vi "Analysis Vol. 3 CSV Read.vi"() -> ()   [LabVIEW 2014] (continued)
2399.01, 2394.29, 2389.45, 2384.42, 2379.46, 2374.5, 2369.85, 2365.32, 2360.97, 2356.55, 2352.38, 2348.17, 2343.81, 2339.36, 2334.89, 2330.02, 2324.83, 2319.71, 2314.4, 2308.87, 2303.33, 2297.78, 2291.87, 2285.95, 2280.16, 2274.42, 2268.74, 2263.33, 2257.96, 2252.44, 2246.89, 2241.34, 2235.57, 2229.67, 2223.7, 2217.56, 2211.19, 2204.8, 2198.33, 2191.78, 2185.2, 2178.68, 2172.08, 2165.53, 2159.12, 2152.93, 2146.84, 2140.86, 2134.88, 2128.82, 2122.54, 2116.07, 2109.39, 2102.62, 2095.88, 2089.08, 2082.34, 2075.72, 2068.95, 2061.64, 2053.63, 2044.73, 2034.67, 2023.62, 2011.78, 1999.41, 1987.03, 1974.65, 1962.27, 1949.9, 1937.52]}, {"Y"=[4.0, 5.0, 6.0, 7.0, 8.0, 9.0, 10.0, 11.0, 12.0, 13.0, 14.0, 15.0, 16.0, 17.0, 18.0, 19.0, 20.0, 21.0, 22.0, 23.0, 24.0, 25.0, 26.0, 27.0, 28.0, 29.0, 30.0, 31.0, 32.0, 33.0, 34.0, 35.0, 36.0, 37.0, 38.0, 39.0, 40.0, 41.0, 42.0, 43.0, 44.0, 45.0, 46.0, 47.0, 48.0, 49.0, 50.0, 51.0, 52.0, 53.0, 54.0, 55.0, 56.0, 57.0, 58.0, 59.0, 60.0, 61.0, 62.0, 63.0, 64.0, 65.0, 66.0, 67.0, 68.0, 69.0, 70.0, 71.0, 72.0, 73.0, 74.0, 75.0, 76.0, 77.0, 78.0, 79.0, 80.0, 81.0, 82.0, 83.0, 84.0, 85.0, 86.0, 87.0, 88.0, 89.0, 90.0, 91.0, 92.0, 93.0, 94.0, 95.0], "Y"=[2494.33, 2488.95, 2483.63, 2478.55, 2473.6, 2468.64, 2463.81, 2458.93, 2454.17, 2449.41, 2444.68, 2439.89, 2435.11, 2430.15, 2425.39, 2420.72, 2416.24, 2411.89, 2407.71, 2403.39, 2399.01, 2394.29, 2389.45, 2384.42, 2379.46, 2374.5, 2369.85, 2365.32, 2360.97, 2356.55, 2352.38, 2348.17, 2343.81, 2339.36, 2334.89, 2330.02, 2324.83, 2319.71, 2314.4, 2308.87, 2303.33, 2297.78, 2291.87, 2285.95, 2280.16, 2274.42, 2268.74, 2263.33, 2257.96, 2252.44, 2246.89, 2241.34, 2235.57, 2229.67, 2223.7, 2217.56, 2211.19, 2204.8, 2198.33, 2191.78, 2185.2, 2178.68, 2172.08, 2165.53, 2159.12, 2152.93, 2146.84, 2140.86, 2134.88, 2128.82, 2122.54, 2116.07, 2109.39, 2102.62, 2095.88, 2089.08, 2082.34, 2075.72, 2068.95, 2061.64, 2053.63, 2044.73, 2034.67, 2023.62, 2011.78, 1999.41, 1987.03, 1974.65, 1962.27, 1949.9, 1937.52]}, {"Y"=[4.0, 5.0, 6.0, 7.0, 8.0, 9.0, 10.0, 11.0, 12.0, 13.0, 14.0, 15.0, 16.0, 17.0, 18.0, 19.0, 20.0, 21.0, 22.0, 23.0, 24.0, 25.0, 26.0, 27.0, 28.0, 29.0, 30.0, 31.0, 32.0, 33.0, 34.0, 35.0, 36.0, 37.0, 38.0, 39.0, 40.0, 41.0, 42.0, 43.0, 44.0, 45.0, 46.0, 47.0, 48.0, 49.0, 50.0, 51.0, 52.0, 53.0, 54.0, 55.0, 56.0, 57.0, 58.0, 59.0, 60.0, 61.0, 62.0, 63.0, 64.0, 65.0, 66.0, 67.0, 68.0, 69.0, 70.0, 71.0, 72.0, 73.0, 74.0, 75.0, 76.0, 77.0, 78.0, 79.0, 80.0, 81.0, 82.0, 83.0, 84.0, 85.0, 86.0, 87.0, 88.0, 89.0, 90.0, 91.0, 92.0, 93.0, 94.0, 95.0], "Y"=[2494.33, 2488.95, 2483.63, 2478.55, 2473.6, 2468.64, 2463.81, 2458.93, 2454.17, 2449.41, 2444.68, 2439.89, 2435.11, 2430.15, 2425.39, 2420.72, 2416.24, 2411.89, 2407.71, 2403.39, 2399.01, 2394.29, 2389.45, 2384.42, 2379.46, 2374.5, 2369.85, 2365.32, 2360.97, 2356.55, 2352.38, 2348.17, 2343.81, 2339.36, 2334.89, 2330.02, 2324.83, 2319.71, 2314.4, 2308.87, 2303.33, 2297.78, 2291.87, 2285.95, 2280.16, 2274.42, 2268.74, 2263.33, 2257.96, 2252.44, 2246.89, 2241.34, 2235.57, 2229.67, 2223.7, 2217.56, 2211.19, 2204.8, 2198.33, 2191.78, 2185.2, 2178.68, 2172.08, 2165.53, 2159.12, 2152.93, 2146.84, 2140.86, 2134.88, 2128.82, 2122.54, 2116.07, 2109.39, 2102.62, 2095.88, 2089.08, 2082.34, 2075.72, 2068.95, 2061.64, 2053.63, 2044.73, 2034.67, 2023.62, 2011.78, 1999.41, 1987.03, 1974.65, 1962.27, 1949.9, 1937.52]}, {"Y"=[4.0, 5.0, 6.0, 7.0, 8.0, 9.0, 10.0, 11.0, 12.0, 13.0, 14.0, 15.0, 16.0, 17.0, 18.0, 19.0, 20.0, 21.0, 22.0, 23.0, 24.0, 25.0, 26.0, 27.0, 28.0, 29.0, 30.0, 31.0, 32.0, 33.0, 34.0, 35.0, 36.0, 37.0, 38.0, 39.0, 40.0, 41.0, 42.0, 43.0, 44.0, 45.0, 46.0, 47.0, 48.0, 49.0, 50.0, 51.0, 52.0, 53.0, 54.0, 55.0, 56.0, 57.0, 58.0, 59.0, 60.0, 61.0, 62.0, 63.0, 64.0, 65.0, 66.0, 67.0, 68.0, 69.0, 70.0, 71.0, 72.0, 73.0, 74.0, 75.0, 76.0, 77.0, 78.0, 79.0, 80.0, 81.0, 82.0, 83.0, 84.0, 85.0, 86.0, 87.0, 88.0, 89.0, 90.0, 91.0, 92.0, 93.0, 94.0, 95.0], "Y"=[2494.33, 2488.95, 2483.63, 2478.55, 2473.6, 2468.64, 2463.81, 2458.93, 2454.17, 2449.41, 2444.68, 2439.89, 2435.11, 2430.15, 2425.39, 2420.72, 2416.24, 2411.89, 2407.71, 2403.39, 2399.01, 2394.29, 2389.45, 2384.42, 2379.46, 2374.5, 2369.85, 2365.32, 2360.97, 2356.55, 2352.38, 2348.17, 2343.81, 2339.36, 2334.89, 2330.02, 2324.83, 2319.71, 2314.4, 2308.87, 2303.33, 2297.78, 2291.87, 2285.95, 2280.16, 2274.42, 2268.74, 2263.33, 2257.96, 2252.44, 2246.89, 2241.34, 2235.57, 2229.67, 2223.7, 2217.56, 2211.19, 2204.8, 2198.33, 2191.78, 2185.2, 2178.68, 2172.08, 2165.53, 2159.12, 2152.93, 2146.84, 2140.86, 2134.88, 2128.82, 2122.54, 2116.07, 2109.39, 2102.62, 2095.88, 2089.08, 2082.34, 2075.72, 2068.95, 2061.64, 2053.63, 2044.73, 2034.67, 2023.62, 2011.78, 1999.41, 1987.03, 1974.65, 1962.27, 1949.9, 1937.52]}, {"Y"=[4.0, 5.0, 6.0, 7.0, 8.0, 9.0, 10.0, 11.0, 12.0, 13.0, 14.0, 15.0, 16.0, 17.0, 18.0, 19.0, 20.0, 21.0, 22.0, 23.0, 24.0, 25.0, 26.0, 27.0, 28.0, 29.0, 30.0, 31.0, 32.0, 33.0, 34.0, 35.0, 36.0, 37.0, 38.0, 39.0, 40.0, 41.0, 42.0, 43.0, 44.0, 45.0, 46.0, 47.0, 48.0, 49.0, 50.0, 51.0, 52.0, 53.0, 54.0, 55.0, 56.0, 57.0, 58.0, 59.0, 60.0, 61.0, 62.0, 63.0, 64.0, 65.0, 66.0, 67.0, 68.0, 69.0, 70.0, 71.0, 72.0, 73.0, 74.0, 75.0, 76.0, 77.0, 78.0, 79.0, 80.0, 81.0, 82.0, 83.0, 84.0, 85.0, 86.0, 87.0, 88.0, 89.0, 90.0, 91.0, 92.0, 93.0, 94.0, 95.0], "Y"=[2494.33, 2488.95, 2483.63, 2478.55, 2473.6, 2468.64, 2463.81, 2458.93, 2454.17, 2449.41, 2444.68, 2439.89, 2435.11, 2430.15, 2425.39, 2420.72, 2416.24, 2411.89, 2407.71, 2403.39, 2399.01, 2394.29, 2389.45, 2384.42, 2379.46, 2374.5, 2369.85, 2365.32, 2360.97, 2356.55, 2352.38, 2348.17, 2343.81, 2339.36, 2334.89, 2330.02, 2324.83, 2319.71, 2314.4, 2308.87, 2303.33, 2297.78, 2291.87, 2285.95, 2280.16, 2274.42, 2268.74, 2263.33, 2257.96, 2252.44, 2246.89, 2241.34, 2235.57, 2229.67, 2223.7, 2217.56, 2211.19, 2204.8, 2198.33, 2191.78, 2185.2, 2178.68, 2172.08, 2165.53, 2159.12, 2152.93, 2146.84, 2140.86, 2134.88, 2128.82, 2122.54, 2116.07, 2109.39, 2102.62, 2095.88, 2089.08, 2082.34, 2075.72, 2068.95, 2061.64, 2053.63, 2044.73, 2034.67, 2023.62, 2011.78, 1999.41, 1987.03, 1974.65, 1962.27, 1949.9, 1937.52]}, {"Y"=[4.0, 5.0, 6.0, 7.0, 8.0, 9.0, 10.0, 11.0, 12.0, 13.0, 14.0, 15.0, 16.0, 17.0, 18.0, 19.0, 20.0, 21.0, 22.0, 23.0, 24.0, 25.0, 26.0, 27.0, 28.0, 29.0, 30.0, 31.0, 32.0, 33.0, 34.0, 35.0, 36.0, 37.0, 38.0, 39.0, 40.0, 41.0, 42.0, 43.0, 44.0, 45.0, 46.0, 47.0, 48.0, 49.0, 50.0, 51.0, 52.0, 53.0, 54.0, 55.0, 56.0, 57.0, 58.0, 59.0, 60.0, 61.0, 62.0, 63.0, 64.0, 65.0, 66.0, 67.0, 68.0, 69.0, 70.0, 71.0, 72.0, 73.0, 74.0, 75.0, 76.0, 77.0, 78.0, 79.0, 80.0, 81.0, 82.0, 83.0, 84.0, 85.0, 86.0, 87.0, 88.0, 89.0, 90.0, 91.0, 92.0, 93.0, 94.0, 95.0], "Y"=[2494.33, 2488.95, 2483.63, 2478.55, 2473.6, 2468.64, 2463.81, 2458.93, 2454.17, 2449.41, 2444.68, 2439.89, 2435.11, 2430.15, 2425.39, 2420.72, 2416.24, 2411.89, 2407.71, 2403.39, 2399.01, 2394.29, 2389.45, 2384.42, 2379.46, 2374.5, 2369.85, 2365.32, 2360.97, 2356.55, 2352.38, 2348.17, 2343.81, 2339.36, 2334.89, 2330.02, 2324.83, 2319.71, 2314.4, 2308.87, 2303.33, 2297.78, 2291.87, 2285.95, 2280.16, 2274.42, 2268.74, 2263.33, 2257.96, 2252.44, 2246.89, 2241.34, 2235.57, 2229.67, 2223.7, 2217.56, 2211.19, 2204.8, 2198.33, 2191.78, 2185.2, 2178.68, 2172.08, 2165.53, 2159.12, 2152.93, 2146.84, 2140.86, 2134.88, 2128.82, 2122.54, 2116.07, 2109.39, 2102.62, 2095.88, 2089.08, 2082.34, 2075.72, 2068.95, 2061.64, 2053.63, 2044.73, 2034.67, 2023.62, 2011.78, 1999.41, 1987.03, 1974.65, 1962.27, 1949.9, 1937.52]}, {"Y"=[4.0, 5.0, 6.0, 7.0, 8.0, 9.0, 10.0, 11.0, 12.0, 13.0, 14.0, 15.0, 16.0, 17.0, 18.0, 19.0, 20.0, 21.0, 22.0, 23.0, 24.0, 25.0, 26.0, 27.0, 28.0, 29.0, 30.0, 31.0, 32.0, 33.0, 34.0, 35.0, 36.0, 37.0, 38.0, 39.0, 40.0, 41.0, 42.0, 43.0, 44.0, 45.0, 46.0, 47.0, 48.0, 49.0, 50.0, 51.0, 52.0, 53.0, 54.0, 55.0, 56.0, 57.0, 58.0, 59.0, 60.0, 61.0, 62.0, 63.0, 64.0, 65.0, 66.0, 67.0, 68.0, 69.0, 70.0, 71.0, 72.0, 73.0, 74.0, 75.0, 76.0, 77.0, 78.0, 79.0, 80.0, 81.0, 82.0, 83.0, 84.0, 85.0, 86.0, 87.0, 88.0, 89.0, 90.0, 91.0, 92.0, 93.0, 94.0, 95.0], "Y"=[2494.33, 2488.95, 2483.63, 2478.55, 2473.6, 2468.64, 2463.81, 2458.93, 2454.17, 2449.41, 2444.68, 2439.89, 2435.11, 2430.15, 2425.39, 2420.72, 2416.24, 2411.89, 2407.71, 2403.39, 2399.01, 2394.29, 2389.45, 2384.42, 2379.46, 2374.5, 2369.85, 2365.32, 2360.97, 2356.55, 2352.38, 2348.17, 2343.81, 2339.36, 2334.89, 2330.02, 2324.83, 2319.71, 2314.4, 2308.87, 2303.33, 2297.78, 2291.87, 2285.95, 2280.16, 2274.42, 2268.74, 2263.33, 2257.96, 2252.44, 2246.89, 2241.34, 2235.57, 2229.67, 2223.7, 2217.56, 2211.19, 2204.8, 2198.33, 2191.78, 2185.2, 2178.68, 2172.08, 2165.53, 2159.12, 2152.93, 2146.84, 2140.86, 2134.88, 2128.82, 2122.54, 2116.07, 2109.39, 2102.62, 2095.88, 2089.08, 2082.34, 2075.72, 2068.95, 2061.64, 2053.63, 2044.73, 2034.67, 2023.62, 2011.78, 1999.41, 1987.03, 1974.65, 1962.27, 1949.9, 1937.52]}, {"Y"=[4.0, 5.0, 6.0, 7.0, 8.0, 9.0, 10.0, 11.0, 12.0, 13.0, 14.0, 15.0, 16.0, 17.0, 18.0, 19.0, 20.0, 21.0, 22.0, 23.0, 24.0, 25.0, 26.0, 27.0, 28.0, 29.0, 30.0, 31.0, 32.0, 33.0, 34.0, 35.0, 36.0, 37.0, 38.0, 39.0, 40.0, 41.0, 42.0, 43.0, 44.0, 45.0, 46.0, 47.0, 48.0, 49.0, 50.0, 51.0, 52.0, 53.0, 54.0, 55.0, 56.0, 57.0, 58.0, 59.0, 60.0, 61.0, 62.0, 63.0, 64.0, 65.0, 66.0, 67.0, 68.0, 69.0, 70.0, 71.0, 72.0, 73.0, 74.0, 75.0, 76.0, 77.0, 78.0, 79.0, 80.0, 81.0, 82.0, 83.0, 84.0, 85.0, 86.0, 87.0, 88.0, 89.0, 90.0, 91.0, 92.0, 93.0, 94.0, 95.0], "Y"=[2494.33, 2488.95, 2483.63, 2478.55, 2473.6, 2468.64, 2463.81, 2458.93, 2454.17, 2449.41, 2444.68, 2439.89, 2435.11, 2430.15, 2425.39, 2420.72, 2416.24, 2411.89, 2407.71, 2403.39, 2399.01, 2394.29, 2389.45, 2384.42, 2379.46, 2374.5, 2369.85, 2365.32, 2360.97, 2356.55, 2352.38, 2348.17, 2343.81, 2339.36, 2334.89, 2330.02, 2324.83, 2319.71, 2314.4, 2308.87, 2303.33, 2297.78, 2291.87, 2285.95, 2280.16, 2274.42, 2268.74, 2263.33, 2257.96, 2252.44, 2246.89, 2241.34, 2235.57, 2229.67, 2223.7, 2217.56, 2211.19, 2204.8, 2198.33, 2191.78, 2185.2, 2178.68, 2172.08, 2165.53, 2159.12, 2152.93, 2146.84, 2140.86, 2134.88, 2128.82, 2122.54, 2116.07, 2109.39, 2102.62, 2095.88, 2089.08, 2082.34, 2075.72, 2068.95, 2061.64, 2053.63, 2044.73, 2034.67, 2023.62, 2011.78, 1999.41, 1987.03, 1974.65, 1962.27, 1949.9, 1937.52]}] caption="Reference plot:"
  in  "Load Dye 2":path=path "C:/Users/labuser/Desktop/Arbeit/Experimental Data/Selection via Gelation Project/2021-05-10 Dorothea meltingcurves/melting curves dna/step 1/melting curves 2021-05-12 -  Melt Curve RFU Results_FAM.csv"
  in  "Reference \non/off":bool=TRUE
  in  "STOP":bool
  out "Dye2withBaselineCorrectio":dbl[][](array[numeric])=[[0.0, 4721.59401069584, 4726.64557983141, 4731.69720585736, 4736.72035903032, 4741.6216490146, 4746.19464965707, 4750.77546264608, 4755.13221756768, 4759.44159755608, 4763.89791396376, 4768.45333576223, 4773.03439707822, 4777.77977396049, 4782.53780205103, 4787.25892226452, 4791.97529358062, 4796.91300937426, 4801.61522170524, 4806.32202250741, 4810.93165344366, 4815.32270660079, 4819.15747599548, 4823.15365637635, 4827.05620435302, 4831.11932397294, 4835.44455829981, 4840.13821284811, 4844.89868237613, 4849.72347270819, 4854.55598974164, 4859.30049974853, 4863.79330506012, 4868.06003683746, 4872.40360247469, 4876.48257410991, 4880.49222398608, 4884.66860430045, 4889.23532566947, 4893.60767815332, 4898.14721099649, 4902.8335972453, 4907.55580598647, 4911.69484044918, 4915.77151333199, 4919.86201149958, 4923.86627488786, 4927.85737755496, 4932.2086278581, 4936.7058924887, 4941.19259968617, 4945.45646686776, 4949.70852542204, 4954.02738779181, 4958.70620656545, 4963.3373268874, 4968.1270371998, 4972.78255793418, 4977.19752478803, 4980.86104806113, 4984.48505580278, 4988.14503964276, 4991.90606946941, 4995.71108454377, 4999.84169025866, 5003.79220065297, 5007.79451836246, 5011.69904254421, 5015.55248715627, 5019.4211520663, 5023.46854922211, 5027.31444684709, 5031.28390945256, 5035.21630010117, 5039.18771534215, 5043.297928556, 5047.28534502707, 5050.97484453209, 5054.58029400532, 5057.9925558248, 5061.03113489723, 5064.19189460972, 5067.37675898951, 5070.55704176141, 5073.65523291141, 5076.76172826201, 5079.69065606831, 5082.68394797735, 5085.57389782356, 5088.5962155605, 5091.68654322026, 5094.89447116713, 5098.12219561475, 5101.43434995644, 5104.58157320642, 5107.8598516264, 5111.36204846851, 5114.81342414506, 5118.78218391394, 5123.03726144675, 5127.41177098768, 5131.74312272957, 5136.39151578824, 5140.39791781123, 5144.63135682615, 5148.75170796368, 5152.93125959229, 5157.09173855716, 5161.70979771955, 5166.02742357914, 5170.41958302151, 5174.69823644507, 5178.76165176852, 5182.86433598839, 5187.08415587395, 5191.40660982161, 5195.97381163606, 5200.69896363319, 5205.2834506216, 5209.82139171157, 5214.016470183, 5217.77454547304, 5221.28564607111, 5224.59798553874, 5227.60049882735, 5230.48504907438, 5233.03480180081, 5235.09586969891]]
  # "Load data in a defined format:"
  # "Data Format:\n* 1st column contain Temperature/Time\n* all the rest columns contain signal of samples"
  # "Select wells, give names, and define concentrations:"
  # "Minutes"
  # "Temperature"
  # "divide all channels by reference channel"
  # "dbr=divided by reference"
  # "nr=no reference"
  # "Graph3 - Michaelis-Menten\n(Needs a fit from Graph2)"
  # "Graph1: Data (+/- ref correction)"
  # "Graph2: Corrections & fits"
  # "(Needs Baseline)"
  # "(Needs Concentrations)"
  # "Vmax"
  # "Km"
  # "Graph4: Turnover Analysis\n(Needs line fit in plateau in Graph2 to adjust concentration)"
  # "Graph3 - Michaelis-Menten\n(Needs a fit from Graph2)"
  # "Graph1: Data (+/- ref correction)"
  # "Graph2: Corrections & fits"
  # "(Needs Baseline)"
  # "(Needs Concentrations)"
  # "Vmax"
  # "Km"
  # "Intercalator"
  # "Quenching"
  # "R=0.0019872041 kcal/(mole*K)"
  # "Constant Concentration"
  # "Dilution"
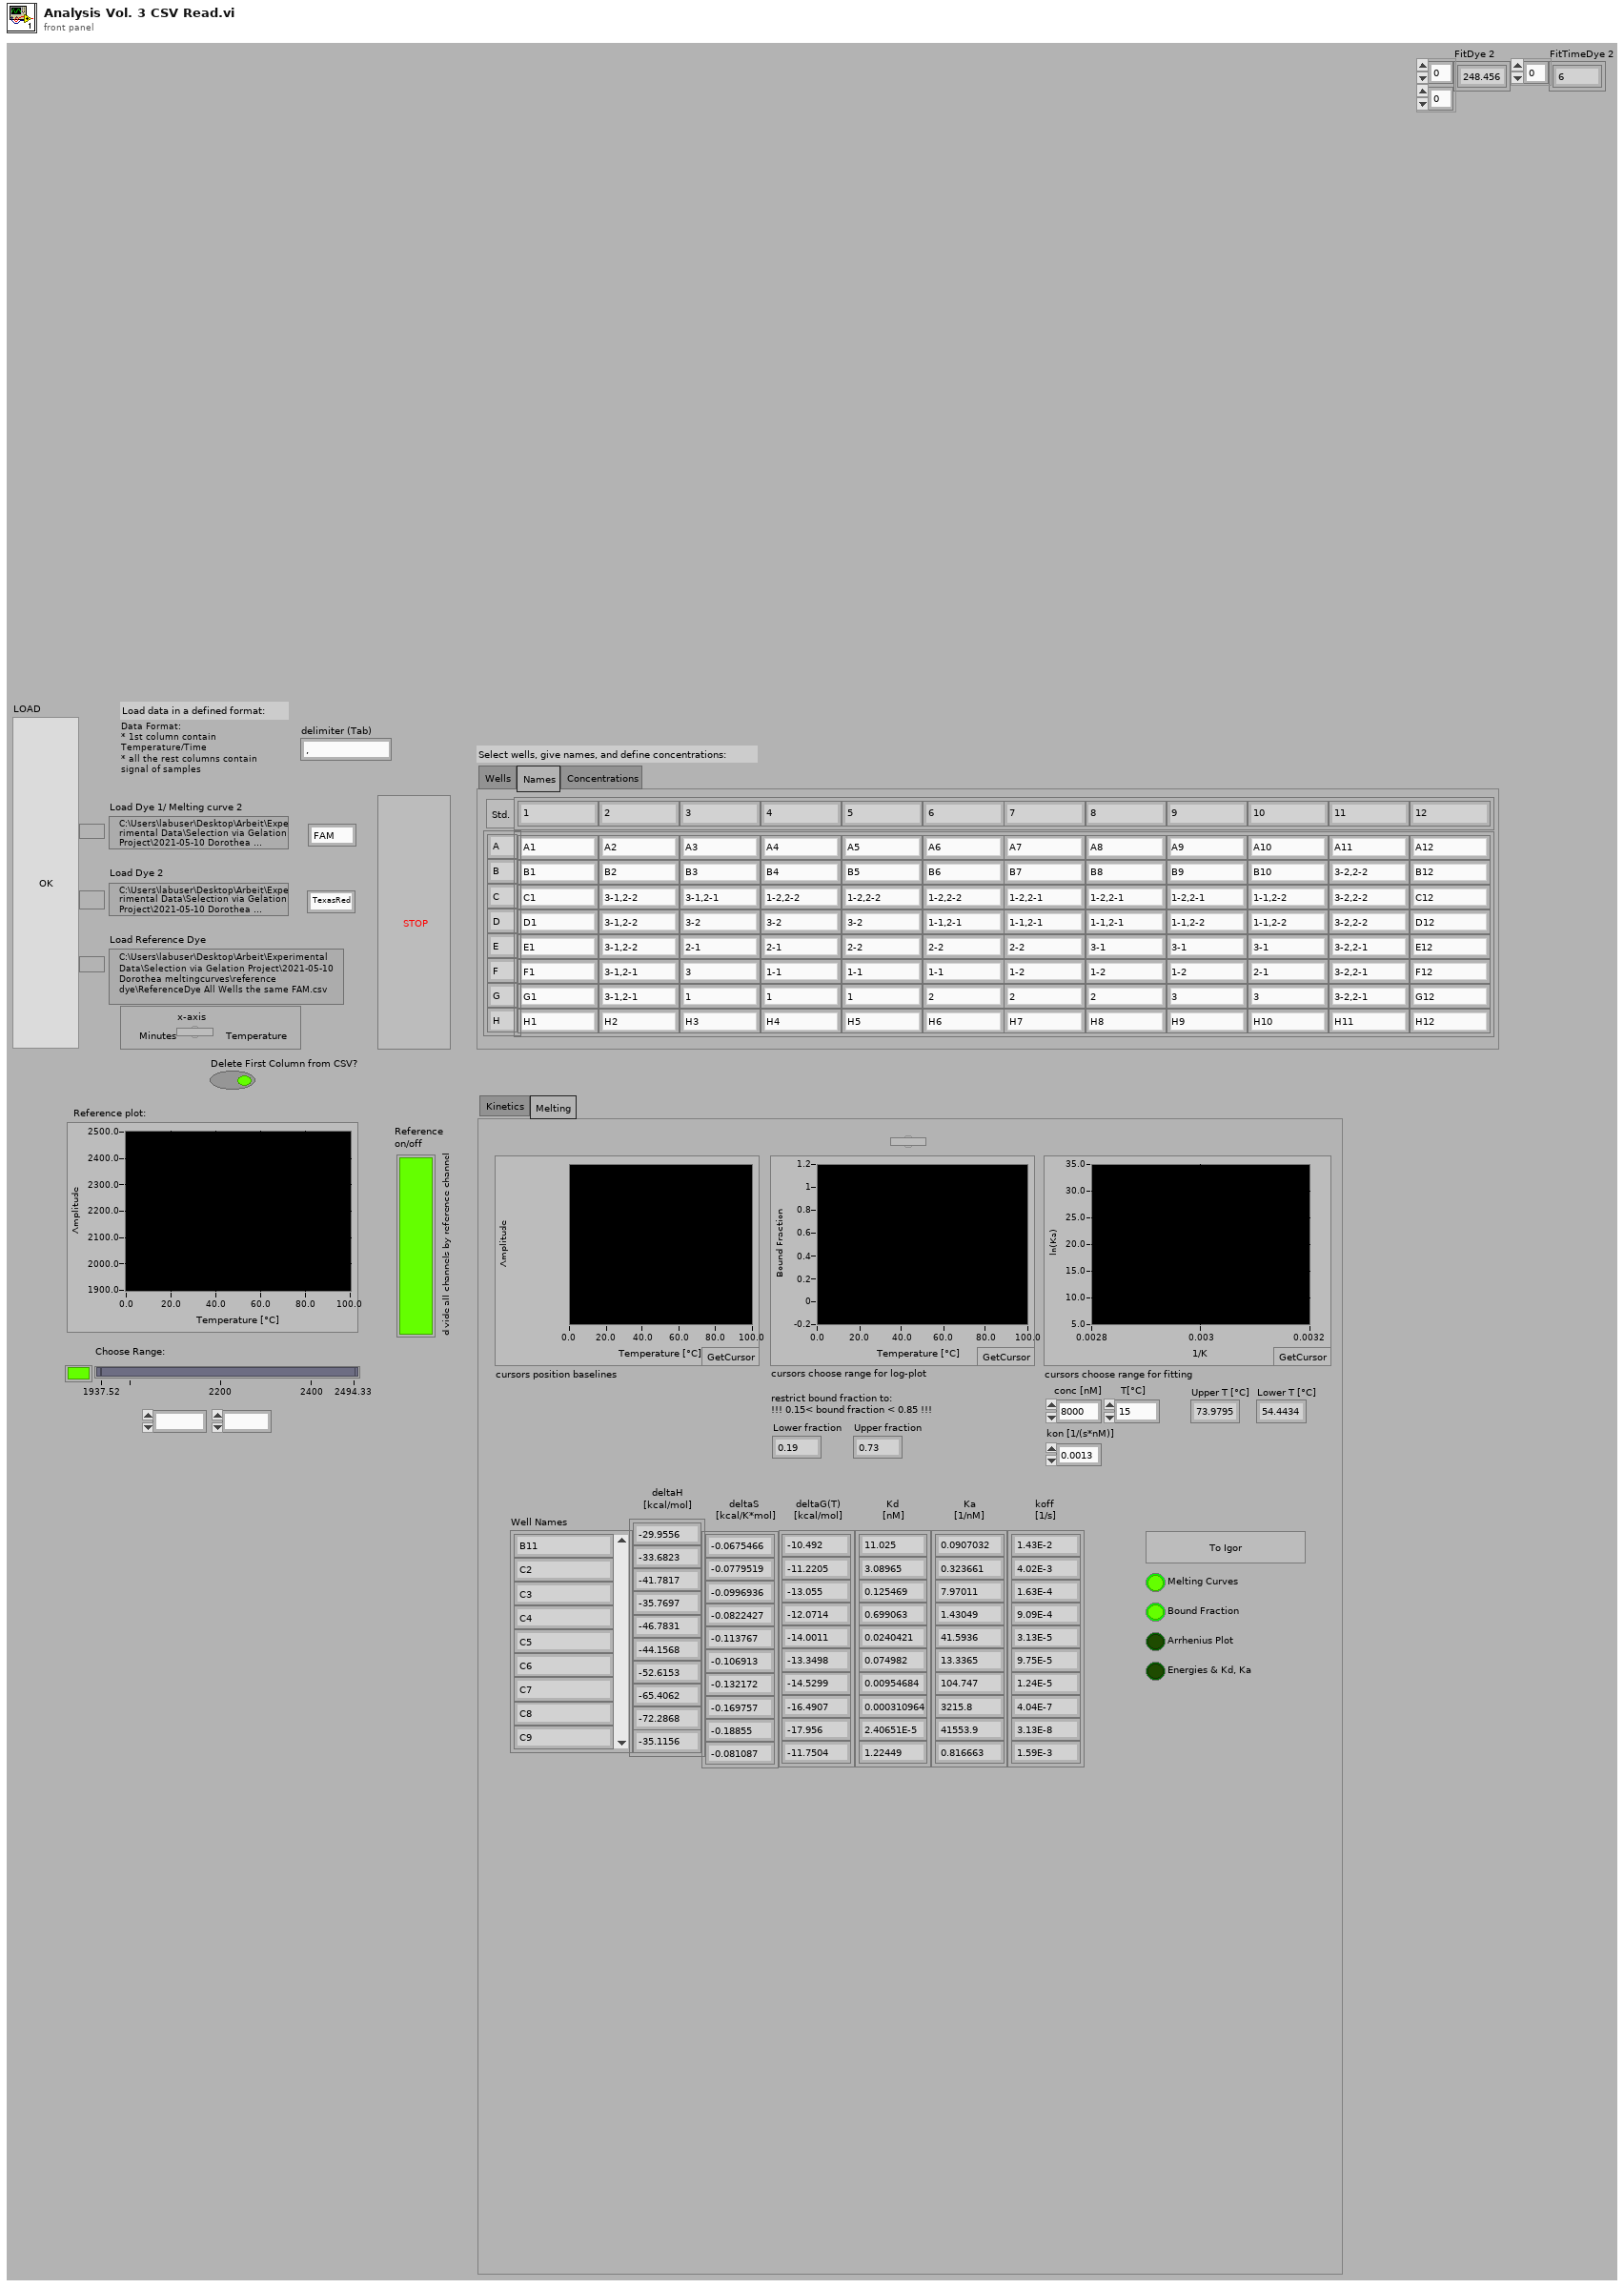
[diagram p1: front panel]
types:
  T1 = cluster{"Concetrations":dbl[], "FitDye1Slopes":dbl[]}[]
  T2 = cluster{"Concetrations":dbl[], "best nonlinear fit":dbl[]}[]
  T3 = cluster{"model":string, "Parameters":string[], "x":string}
  T4 = cluster{"Temp/Time\nranged":dbl[], "Dye1/Melting ranged":dbl[]}
  T5 = cluster{"Concetrations":dbl[], "FitDye1Slopes":dbl[]}
  T6 = cluster{"Concetrations":dbl[], "best nonlinear fit":dbl[]}
  T7 = cluster{"Concetrations":dbl[], "FitDye2Slopes":dbl[]}
  T8 = cluster{"Concetrations":dbl[], "FitDye2Slopes":dbl[]}[]
  T9 = cluster{"Temp/Time\nranged":dbl[], "Dye2 ranged":dbl[]}
  T10 = cluster{"Temp/Time":dbl[], "Dye 1/Melting":dbl[]}
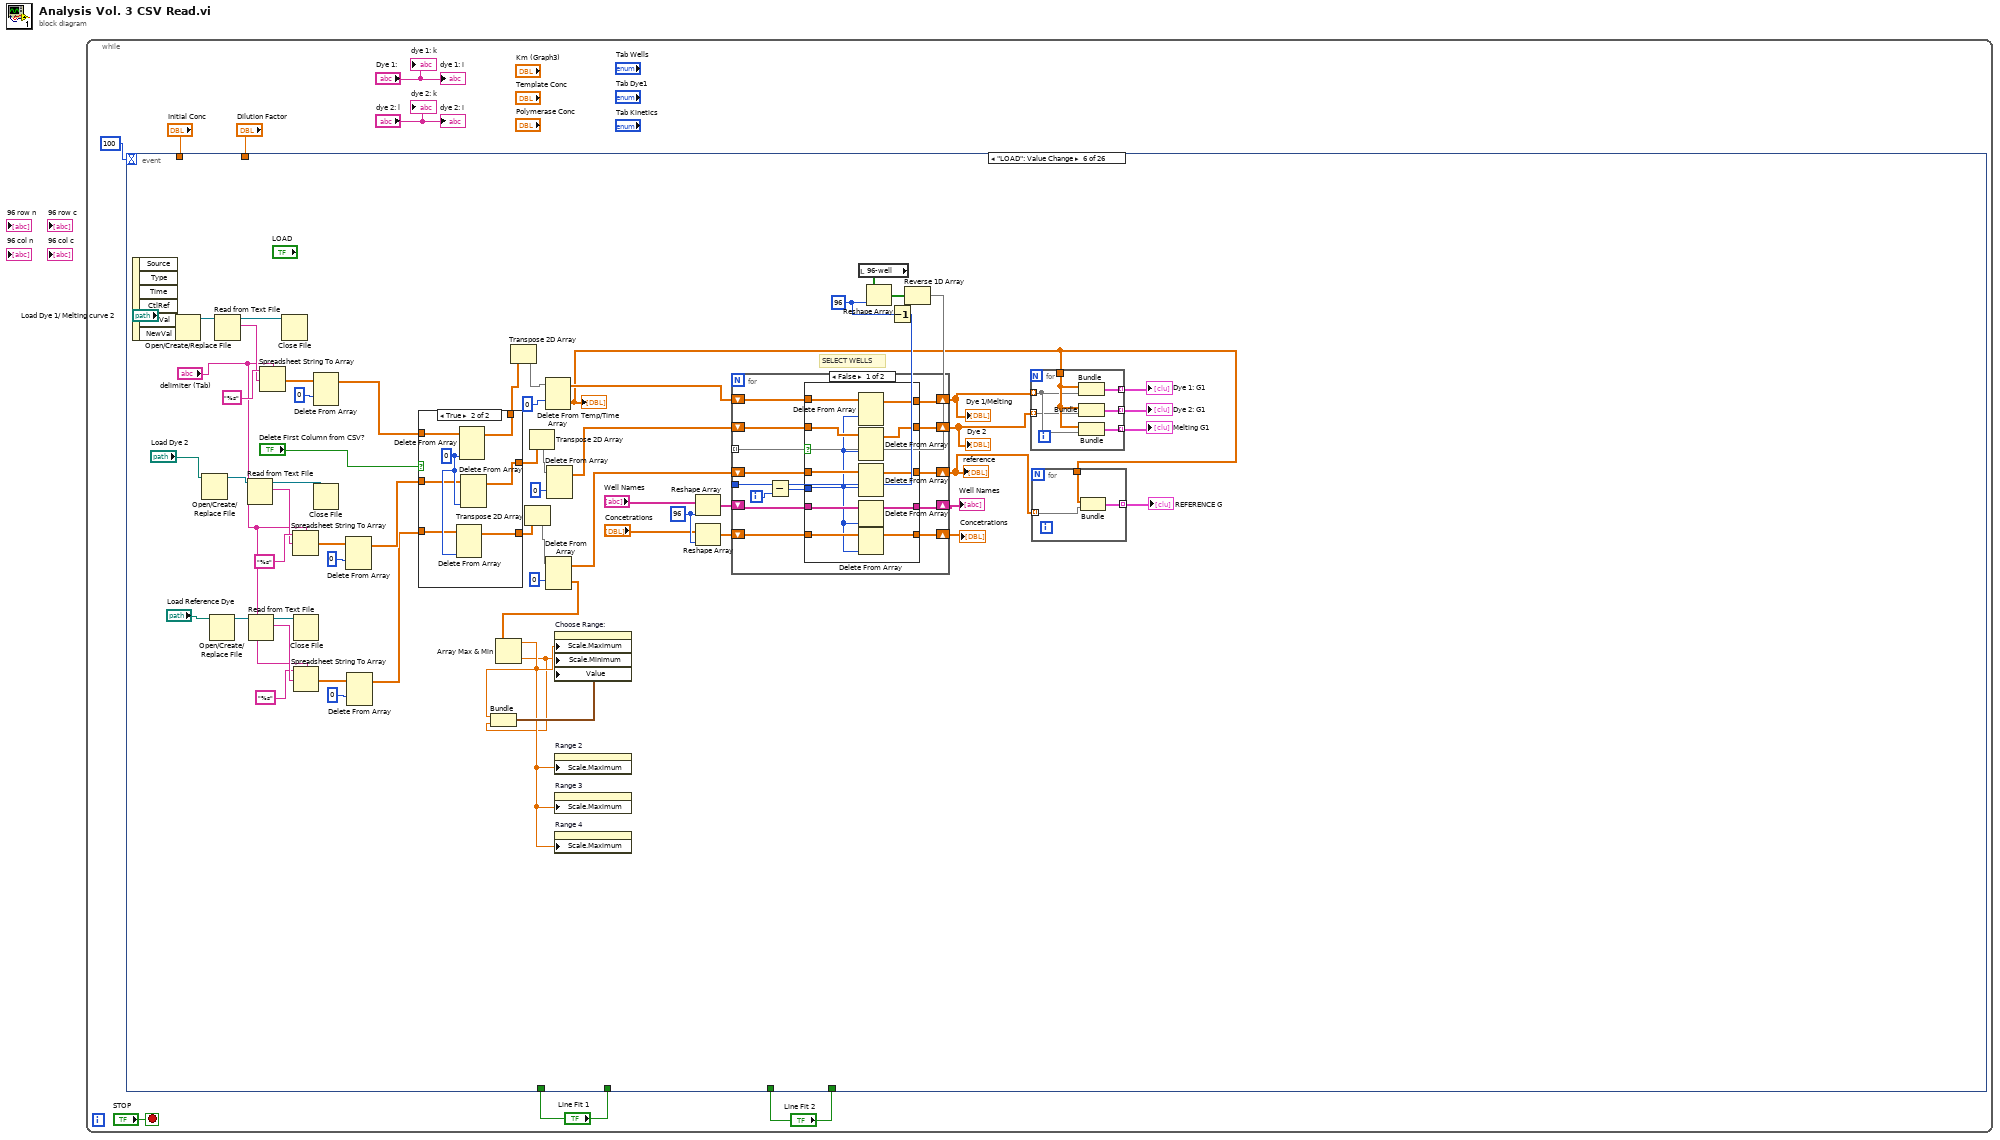
[diagram p0: block diagram]
diagram:
  n1 = while {
    stop <- "STOP" stop-if-true
    n2 = event shown="[5] \"LOAD\": Value Change" {
      selector: _ -> [_ _ _ _ _ _ _ _ _ _ _ _ _ _ _ _ _ _ _ _ _ _ _ _ _ _]
      dyn-events: _ -> [_ _ _ _ _ _ _ _ _ _ _ _ _ _ _ _ _ _ _ _ _ _ _ _ _ _]
      timeout: 100 -> [_ _ _ _ _ _ _ _ _ _ _ _ _ _ _ _ _ _ _ _ _ _ _ _ _ _]
      tunnel: "Initial Conc" -> [_ _ _ _ _ _ _ _ _ _ _ _ _ _ _ _ _ _ _ _ _ _ _ w980 w997 _]
      tunnel: "Dilution Factor" -> [_ _ _ _ _ _ _ _ _ _ _ _ _ _ _ _ _ _ _ _ _ _ _ w979 w996 _]
      tunnel: "Line Fit 1" -> [_ _ _ _ _ _ _ _ _ _ _ _ _ _ _ w616 _ _ _ _ _ _ _ _ _ _]
      tunnel: "Line Fit 2" -> [_ _ _ _ _ _ _ _ _ _ _ _ _ _ _ _ _ _ _ w828 _ _ _ _ _ _]
      tunnel: "Line Fit 1" -> [_ w21 _ _ _ _ _ _ _ _ _ _ _ _ _ _ _ _ _ _ _ _ _ _ _ _]
      tunnel: "Line Fit 2" -> [_ w20 _ _ _ _ _ _ _ _ _ _ _ _ _ _ _ _ _ _ _ _ _ _ _ _]
      event Timeout {
        n3 = event-data() -> ()  [unwired: 1 in, 1 out]
      }
      event "To Igor": Value Change {
        n4 = event-data() -> ("NewVal"=w22:bool)  [unwired: 1 in]
        n5 = local read "Temp/Time\nranged"() -> (w17:dbl[])
        n6 = local read "Dye1/Melting ranged"() -> (w16:dbl[][])
        n7 = local read "Dye2 ranged"() -> (w15:dbl[][])
        n8 = case shown="True" w22 {
          tunnel: w17 -> [_ w26]
          tunnel: "DY530" -> [_ w39]
          tunnel: "FAM" -> [_ w38]
          tunnel: w16 -> [_ w37]
          tunnel: w15 -> [_ w36]
          tunnel: "Dye2: G2" -> [_ w35]
          tunnel: "Dye1: G2" -> [_ w23]
          tunnel: "Dye1: G1" -> [_ w30]
          tunnel: "Dye2: G1" -> [_ w29]
          tunnel: "Dye1: G3" -> [_ w28]
          tunnel: "Dye2: G3" -> [_ w27]
          tunnel: w21 -> [_ w25]
          tunnel: w20 -> [_ w24]
          frame False {
          }
          frame True {
            n9 = local read "Reference \non/off"() -> (w32:bool)
            n10 = Select(t="_dbr_" ("string"), s=w32, f="_nr_" ("string")) -> (s? t:f=w31:string)
            n11 = case shown="True" w39 {
              tunnel: w36 -> [_ w48]
              tunnel: w35 -> [_ w45]
              tunnel: w31 -> [_ w47]
              tunnel: w29 -> [_ w46]
              tunnel: w27 -> [_ w43]
              tunnel: w26 -> [_ w42]
              tunnel: w24 -> [_ w40]
              frame False {
              }
              frame True {
                n12 = call "1D_Data_to_Igor.vi"("Wave Name"="Minutes" ("string"), "Data"=w42) -> ()  [unwired: 9 in, 1 out]
                n13 = local read "dye 2: l"() -> (w44:string)
                n14 = case shown="True" w45 {
                  tunnel: w44 -> [_ w88]
                  tunnel: w47 -> [_ w87]
                  frame False {
                  }
                  frame True {
                    n15 = local read "Dye2withBaselineCorrectio"() -> (w89:dbl[][])
                    n16 = local read "Well Names"() -> (w86:string[])
                    n17 = for {
                      tunnel: w89 -> [w95] mode=indexing
                      tunnel: w88 -> [w93]
                      tunnel: w87 -> [w92]
                      tunnel: w86 -> [w91] mode=indexing
                      n18 = Concatenate Strings(w93, w92, "graph2_" ("string"), w91) -> (w94:string)
                      n19 = call "1D_Data_to_Igor.vi"("Wave Name"=w94, "Data"=w95) -> ()  [unwired: 9 in, 1 out]
                    }
                  }
                }
                n20 = case shown="True" w46 {
                  tunnel: w48 -> [_ w80]
                  tunnel: w44 -> [_ w79]
                  tunnel: w47 -> [_ w78]
                  frame False {
                  }
                  frame True {
                    n21 = local read "Well Names"() -> (w77:string[])
                    n22 = for {
                      tunnel: w80 -> [w85] mode=indexing
                      tunnel: w79 -> [w84]
                      tunnel: w78 -> [w82]
                      tunnel: w77 -> [w81] mode=indexing
                      n23 = Concatenate Strings(w84, w82, w81) -> (w83:string)
                      n24 = call "1D_Data_to_Igor.vi"("Wave Name"=w83, "Data"=w85) -> ()  [unwired: 9 in, 1 out]
                    }
                  }
                }
                n25 = case shown="True" w45 {
                  tunnel: w44 -> [_ w64]
                  tunnel: w40 -> [_ w63]
                  frame False {
                  }
                  frame True {
                    n26 = case shown="True" w63 {
                      tunnel: w64 -> [_ w67]
                      frame False {
                      }
                      frame True {
                        # "True=\nFits will be exported"
                        n27 = local read "FitDye 2"() -> (w65:dbl[][])
                        n28 = local read "Well Names"() -> (w68:string[])
                        n29 = for {
                          tunnel: w65 -> [w76] mode=indexing
                          tunnel: w68 -> [w74] mode=indexing
                          tunnel: w67 -> [w71]
                          tunnel: "_fit_" ("string") -> [w73]
                          n30 = local read "FitTimeDye 2"() -> (w69:dbl[])
                          n31 = Concatenate Strings(w71, "_fit_time" ("string")) -> (w72:string)
                          n32 = Concatenate Strings(w71, w73, w74) -> (w75:string)
                          n33 = call "1D_Data_to_Igor.vi"("Wave Name"=w72, "Data"=w69) -> ()  [unwired: 9 in, 1 out]
                          n34 = call "1D_Data_to_Igor.vi"("Wave Name"=w75, "Data"=w76) -> ()  [unwired: 9 in, 1 out]
                        }
                      }
                    }
                  }
                }
                n35 = case shown="True" w43 {
                  tunnel: w44 -> [_ w51]
                  frame False {
                  }
                  frame True {
                    n36 = local read "SlopesDye2"() -> (w58:dbl[])
                    n37 = local read "ConcentrationDye2"() -> (w59:dbl[])
                    n38 = local read "best nonlinear fit Dye2"() -> (w54:dbl[])
                    n39 = Concatenate Strings(w51, "Sample Name 2", "_Conc" ("string")) -> (w49:string)
                    n40 = Concatenate Strings(w51, "Sample Name 2", "_Rate" ("string")) -> (w62:string)
                    n41 = call "1D_Data_to_Igor.vi"("Wave Name"=w49, "Data"=w59) -> ()  [unwired: 9 in, 1 out]
                    n42 = call "1D_Data_to_Igor.vi"("Wave Name"=w62, "Data"=w58) -> ()  [unwired: 9 in, 1 out]
                    n43 = local read "best fit parameters 1"() -> (w57:dbl[])
                    n44 = Concatenate Strings(w51, "Sample Name 2", "_Vmax_Km" ("string")) -> (w56:string)
                    n45 = call "1D_Data_to_Igor.vi"("Wave Name"=w56, "Data"=w57) -> ()  [unwired: 9 in, 1 out]
                    n46 = Concatenate Strings(w51, "Sample Name 2", "_Fit" ("string")) -> (w50:string)
                    n47 = call "1D_Data_to_Igor.vi"("Wave Name"=w50, "Data"=w54) -> ()  [unwired: 9 in, 1 out]
                  }
                }
              }
            }
            n48 = case shown="True" w38 {
              tunnel: w37 -> [_ w104]
              tunnel: w23 -> [_ w96]
              tunnel: w31 -> [_ w103]
              tunnel: w30 -> [_ w102]
              tunnel: w28 -> [_ w101]
              tunnel: w26 -> [_ w98]
              tunnel: w25 -> [_ w97]
              frame False {
              }
              frame True {
                n49 = local read "Dye 1:"() -> (w100:string)
                n50 = call "1D_Data_to_Igor.vi"("Wave Name"="Minutes" ("string"), "Data"=w98) -> ()  [unwired: 9 in, 1 out]
                n51 = case shown="True" w96 {
                  tunnel: w100 -> [_ w144]
                  tunnel: w103 -> [_ w142]
                  frame False {
                  }
                  frame True {
                    n52 = local read "Dye1withBaselineCorrection"() -> (w145:dbl[][])
                    n53 = local read "Well Names"() -> (w143:string[])
                    n54 = for {
                      tunnel: w145 -> [w151] mode=indexing
                      tunnel: w144 -> [w149]
                      tunnel: w143 -> [w147] mode=indexing
                      tunnel: w142 -> [w148]
                      n55 = Concatenate Strings(w149, w148, "graph2_" ("string"), w147) -> (w150:string)
                      n56 = call "1D_Data_to_Igor.vi"("Wave Name"=w150, "Data"=w151) -> ()  [unwired: 9 in, 1 out]
                    }
                  }
                }
                n57 = case shown="True" w102 {
                  tunnel: w104 -> [_ w136]
                  tunnel: w100 -> [_ w134]
                  tunnel: w103 -> [_ w133]
                  frame False {
                  }
                  frame True {
                    n58 = local read "Well Names"() -> (w135:string[])
                    n59 = for {
                      tunnel: w136 -> [w141] mode=indexing
                      tunnel: w135 -> [w137] mode=indexing
                      tunnel: w134 -> [w139]
                      tunnel: w133 -> [w138]
                      n60 = Concatenate Strings(w139, w138, w137) -> (w140:string)
                      n61 = call "1D_Data_to_Igor.vi"("Wave Name"=w140, "Data"=w141) -> ()  [unwired: 9 in, 1 out]
                    }
                  }
                }
                n62 = case shown="True" w96 {
                  tunnel: w100 -> [_ w120]
                  tunnel: w97 -> [_ w119]
                  frame False {
                  }
                  frame True {
                    n63 = case shown="True" w119 {
                      tunnel: w120 -> [_ w123]
                      frame False {
                      }
                      frame True {
                        # "True=\nFits will be exported"
                        n64 = local read "Well Names"() -> (w124:string[])
                        n65 = local read "FitDye1"() -> (w122:dbl[][])
                        n66 = for {
                          tunnel: w122 -> [w132] mode=indexing
                          tunnel: w124 -> [w130] mode=indexing
                          tunnel: w123 -> [w126]
                          tunnel: "_fit_" ("string") -> [w129]
                          n67 = local read "FitTimeDye1"() -> (w128:dbl[])
                          n68 = Concatenate Strings(w126, "_fit_time" ("string")) -> (w127:string)
                          n69 = Concatenate Strings(w126, w129, w130) -> (w131:string)
                          n70 = call "1D_Data_to_Igor.vi"("Wave Name"=w127, "Data"=w128) -> ()  [unwired: 9 in, 1 out]
                          n71 = call "1D_Data_to_Igor.vi"("Wave Name"=w131, "Data"=w132) -> ()  [unwired: 9 in, 1 out]
                        }
                      }
                    }
                  }
                }
                n72 = case shown="True" w101 {
                  tunnel: w100 -> [_ w107]
                  frame False {
                  }
                  frame True {
                    n73 = local read "ConcentrationDye1"() -> (w115:dbl[])
                    n74 = local read "SlopesDye1"() -> (w114:dbl[])
                    n75 = Concatenate Strings(w107, "Sample Name", "_Conc" ("string")) -> (w105:string)
                    n76 = Concatenate Strings(w107, "Sample Name", "_Rate" ("string")) -> (w118:string)
                    n77 = local read "best nonlinear fit Dye1"() -> (w110:dbl[])
                    n78 = call "1D_Data_to_Igor.vi"("Wave Name"=w105, "Data"=w115) -> ()  [unwired: 9 in, 1 out]
                    n79 = call "1D_Data_to_Igor.vi"("Wave Name"=w118, "Data"=w114) -> ()  [unwired: 9 in, 1 out]
                    n80 = local read "best fit parameters 2"() -> (w113:dbl[])
                    n81 = Concatenate Strings(w107, "Sample Name", "_Vmax_Km" ("string")) -> (w112:string)
                    n82 = Concatenate Strings(w107, "Sample Name", "_Fit" ("string")) -> (w106:string)
                    n83 = call "1D_Data_to_Igor.vi"("Wave Name"=w112, "Data"=w113) -> ()  [unwired: 9 in, 1 out]
                    n84 = call "1D_Data_to_Igor.vi"("Wave Name"=w106, "Data"=w110) -> ()  [unwired: 9 in, 1 out]
                  }
                }
              }
            }
          }
        }
      }
      event "GetCursor: melting G1": Value Change {
        n85 = event-data() -> ()  [unwired: 1 in, 1 out]
        n86 = property on="Melting G1" class="XYGraph (strict)"() -> ("XScale.Minimum"=w153:dbl, "XScale.Maximum"=w156:dbl)  [unwired: 2 in, 2 out]
        n87 = Subtract(x=w156, y=w153) -> (x-y=w158:dbl)
        n88 = Divide(x=w158, y=2.0) -> (x/y=w154:dbl)
        n89 = Add(x=w153, y=w154) -> (x+y=w155:dbl)
        n90 = property on="Melting G1" class="XYGraph (strict)"("Active Cursor"=u32 0, "Cursor.Cursor X"=w155) -> ()  [unwired: 2 in, 2 out]
        n91 = property on="Melting G1" class="XYGraph (strict)"("Active Cursor"=u32 1, "Cursor.Cursor X"=w155) -> ()  [unwired: 2 in, 2 out]
        n92 = property on="Melting G1" class="XYGraph (strict)"("Active Cursor"=u32 2, "Cursor.Cursor X"=w155) -> ()  [unwired: 2 in, 2 out]
        n93 = property on="Melting G1" class="XYGraph (strict)"("Active Cursor"=u32 3, "Cursor.Cursor X"=w155) -> ()  [unwired: 2 in, 2 out]
        n94 = local read "Intercalating/\nQuenching"() -> (w152:bool)
        n95 = property on="Intercalating/\nQuenching" class="Bool (strict)"("Val(Sgnl)"=w152) -> ()  [unwired: 2 in, 2 out]
      }
      event "GetCursor: melting G2": Value Change {
        n96 = event-data() -> ()  [unwired: 1 in, 1 out]
        n97 = property on="Melting G2" class="XYGraph (strict)"() -> ("XScale.Minimum"=w164:dbl, "XScale.Maximum"=w169:dbl)  [unwired: 2 in, 2 out]
        n98 = Subtract(x=w169, y=w164) -> (x-y=w170:dbl)
        n99 = Divide(x=w170, y=2.0) -> (x/y=w165:dbl)
        n100 = Add(x=w164, y=w165) -> (x+y=w166:dbl)
        n101 = property on="Melting G2" class="XYGraph (strict)"("Active Cursor"=u32 0, "Cursor.Cursor X"=w166) -> ()  [unwired: 2 in, 2 out]
        n102 = property on="Melting G2" class="XYGraph (strict)"("Active Cursor"=u32 1, "Cursor.Cursor X"=w166) -> ()  [unwired: 2 in, 2 out]
        n103 = local read "Intercalating/\nQuenching"() -> (w163:bool)
        n104 = property on="Intercalating/\nQuenching" class="Bool (strict)"("Val(Sgnl)"=w163) -> ()  [unwired: 2 in, 2 out]
      }
      event "GetCursor: melting G3": Value Change {
        n105 = event-data() -> ()  [unwired: 1 in, 1 out]
        n106 = property on="Melting: G3" class="XYGraph (strict)"() -> ("XScale.Minimum"=w172:dbl, "XScale.Maximum"=w177:dbl)  [unwired: 2 in, 2 out]
        n107 = Subtract(x=w177, y=w172) -> (x-y=w178:dbl)
        n108 = Divide(x=w178, y=2.0) -> (x/y=w173:dbl)
        n109 = Add(x=w172, y=w173) -> (x+y=w174:dbl)
        n110 = property on="Melting: G3" class="XYGraph (strict)"("Active Cursor"=u32 0, "Cursor.Cursor X"=w174) -> ()  [unwired: 2 in, 2 out]
        n111 = property on="Melting: G3" class="XYGraph (strict)"("Active Cursor"=u32 1, "Cursor.Cursor X"=w174) -> ()  [unwired: 2 in, 2 out]
      }
      event "LOAD": Value Change {
        w227 = 96 ("dimension size")
        w221 = 96 ("dimension size")
        # "SELECT WELLS"
        n112 = event-data() -> ()  [unwired: 1 in, 6 out]
        n113 = Open/Create/Replace File(file path (use dialog)="Load Dye 1/ Melting curve 2") -> (refnum out=w206:refnum<file>)  [unwired: 5 in, 2 out]
        n114 = Open/Create/Replace File(file path (use dialog)="Load Dye 2") -> (refnum out=w193:refnum<file>)  [unwired: 5 in, 2 out]
        n115 = Open/Create/Replace File(file path (use dialog)="Load Reference Dye") -> (refnum out=w203:refnum<file>)  [unwired: 5 in, 2 out]
        n116 = Read from Text File(file (use dialog)=w206) -> (refnum out=w207:refnum<file>, text=w208:string)  [unwired: 3 in, 2 out]
        n117 = Read from Text File(file (use dialog)=w193) -> (refnum out=w191:refnum<file>, text=w194:string)  [unwired: 3 in, 2 out]
        n118 = Read from Text File(file (use dialog)=w203) -> (refnum out=w202:refnum<file>, text=w201:string)  [unwired: 3 in, 2 out]
        n119 = Spreadsheet String To Array(delimiter (Tab)="delimiter (Tab)", format string="%s", spreadsheet string=w208) -> (array=w210:dbl[][])  [unwired: 1 in]
        n120 = Close File(refnum=w207) -> ()  [unwired: 1 in, 2 out]
        n121 = Spreadsheet String To Array(delimiter (Tab)="delimiter (Tab)", format string="%s", spreadsheet string=w194) -> (array=w196:dbl[][])  [unwired: 1 in]
        n122 = Close File(refnum=w202) -> ()  [unwired: 1 in, 2 out]
        n123 = Spreadsheet String To Array(delimiter (Tab)="delimiter (Tab)", format string="%s", spreadsheet string=w201) -> (array=w199:dbl[][])  [unwired: 1 in]
        n124 = Delete From Array(array=w210, index (row)=0) -> (array with subset deleted=w190:dbl[][])  [unwired: 2 in, 1 out]
        n125 = Close File(refnum=w191) -> ()  [unwired: 1 in, 2 out]
        n126 = Delete From Array(array=w196, index (row)=0) -> (array with subset deleted=w189:dbl[][])  [unwired: 2 in, 1 out]
        n127 = Delete From Array(array=w199, index (row)=0) -> (array with subset deleted=w188:dbl[][])  [unwired: 2 in, 1 out]
        n128 = case shown="True" "Delete First Column from CSV?" {
          tunnel: w189 -> [w243 w250]
          tunnel: w190 -> [w244 w249]
          tunnel: w188 -> [w242 w248]
          tunnel: [w242 w247] -> w181
          tunnel: [w243 w246] -> w182
          tunnel: [w244 w245] -> w184
          frame False {
          }
          frame True {
            w251 = 0 ("index (col)")
            n129 = Delete From Array(array=w248, index (col)=w251) -> (array with subset deleted=w247:dbl[][])  [unwired: 2 in, 1 out]
            n130 = Delete From Array(array=w249, index (col)=w251) -> (array with subset deleted=w245:dbl[][])  [unwired: 2 in, 1 out]
            n131 = Delete From Array(array=w250, index (col)=w251) -> (array with subset deleted=w246:dbl[][])  [unwired: 2 in, 1 out]
          }
        }
        n132 = Transpose 2D Array(2D array=w184) -> (transposed array=w185:dbl[][])
        n133 = Transpose 2D Array(2D array=w181) -> (transposed array=w180:dbl[][])
        n134 = Transpose 2D Array(2D array=w182) -> (transposed array=w183:dbl[][])
        n135 = Delete From Array(array=w185, index (row)=0 ("disabled index (col)")) -> (deleted portion=w216:dbl[], array with subset deleted=w234:dbl[][])  [unwired: 2 in]
        "Temp/Time" <- w216
        n136 = Delete From Array(array=w180, index (row)=0 ("disabled index (col)")) -> (deleted portion=w235:dbl[], array with subset deleted=w218:dbl[][])  [unwired: 2 in]
        n137 = Array Max & Min(array=w235) -> (max value=w213:dbl, min value=w212:dbl)  [unwired: 2 out]
